vi "TimingFunctions_convertToUtcTimestamp.vi"(1 "Time":timestamp) -> (15 "UtcTime":timestamp format="%^<%H:%M:%S%3u %p\n%d/%m/%Y>T")   [LabVIEW 2016]
doc: "Wandelt den Timestamp in UTC um.\n\n11.3.15 / sige"
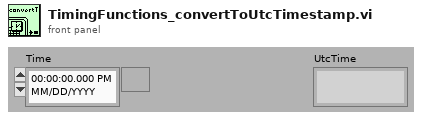
[diagram p1: front panel]
types:
  T1 = typedef "LVDateTimeRec.ctl" = cluster{"fractional second":dbl, "second":i32, "minute":i32, "hour":i32, "day of month":i32, "month":i32, "year":i32, "day of week":i32, "day of year":i32, "DST":i32}
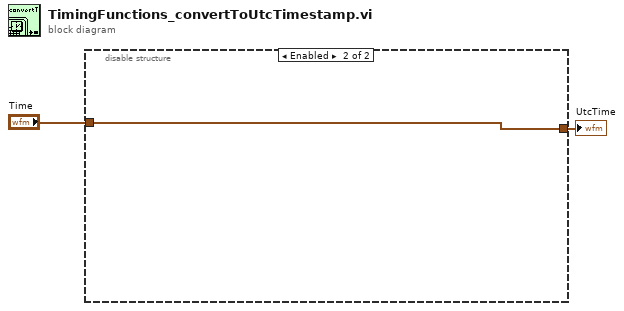
[diagram p0: block diagram]
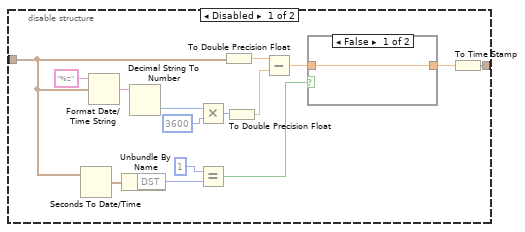
[diagram p2: hidden frame]
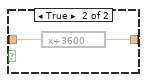
[diagram p3: hidden frame]
diagram:
  n1 = disable-structure shown="Enabled" {
    disable-tunnel: "Time" -> [w4 w21]
    disable-tunnel: [w3 w21] -> w1
    frame Disabled {
      n2 = Seconds To Date/Time(time stamp (now)=w4) -> (date time rec=w10:T1)  [unwired: 1 in]
      n3 = Format Date/Time String(time format string (%c)="%z", seconds (now)=w4) -> (date/time string=w12:string)  [unwired: 1 out]
      n4 = Unbundle By Name(w10) -> ("DST"=w9:i32)
      n5 = Decimal String To Number(string=w12) -> (number=w11:i32)  [unwired: 3 out]
      n6 = Multiply(x=w11, y=3600) -> (x*y=w15:i32)
      n7 = Equal?(x=1, y=w9) -> (x = y?=w7:bool)
      n8 = To Double Precision Float(number=w4) -> (double precision float=w14:dbl)
      n9 = To Double Precision Float(number=w15) -> (double precision float=w13:dbl)
      n10 = Subtract(x=w14, y=w13) -> (x-y=w6:dbl)
      n11 = case shown="False" w7 {
        tunnel: w6 -> [w18 w20]
        tunnel: [w18 w19] -> w5
        frame False {
        }
        frame True {
          n12 = expression code="x+3600"(w20) -> (w19:dbl)
        }
      }
      n13 = To Time Stamp(1:w5) -> (0:w3:timestamp)
    }
    frame Enabled {
    }
  }
  "UtcTime" <- w1
